vi "Begin.vi"(8 "error in":errorcluster) -> (0 "error out":errorcluster)   [LabVIEW 2017]
doc: "Called before other user functions, this VI is expected to open initial I/O refnums, load in file data, and do all program initialization. Notice that the <B>error out</B> terminal is simply used for data flow. Wiring it to other structures or subVIs ensures that this VI runs first."
uses:
  <vilib>/Rock Robotics/WPI/DriverStation/WPI_DriverStationRobotMode2.ctl
  <vilib>/Rock Robotics/WPI/Joystick/WPI_JoystickDeviceEnum.ctl
  <vilib>/Rock Robotics/WPI/ThirdParty/Phoenix-LabVIEW/Motor Controller/Controls/CTRE_Phoenix_MotorControl_ControlMode.ctl
  <vilib>/Rock Robotics/WPI/Solenoid/WPI_SolenoidChannel.ctl
  Robot Global Data.vi
  <vilib>/Rock Robotics/Network Tables/NT Write String Array.vi
  Public/Documents/Cross The Road Electronics/Phoenix-LabVIEW/Pigeon IMU/CTRE_PigeonIMU_Open_TalonSRX.vi
  <vilib>/Rock Robotics/WPI/Solenoid/WPI_SolenoidOpenDouble.vi
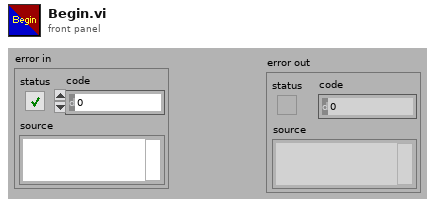
[diagram p1: front panel]
types:
  T1 = typedef "WPI_SolenoidChannel.ctl" = enum8{"Solenoid 0", "Solenoid 1", "Solenoid 2", "Solenoid 3", "Solenoid 4", "Solenoid 5", "Solenoid 6", "Solenoid 7", "Invalid"}
  T2 = typedef "CTRE_Phoenix_MotorControl_ControlMode.ctl" = u16
  T3 = typedef "WPI_JoystickDeviceEnum.ctl" = enum16{"USB 0", "USB 1", "USB 2", "USB 3", "USB 4", "USB 5"}
  T4 = typedef "WPI_DriverStationRobotMode2.ctl" = enum16{"Autonomous Disabled", "Autonomous Enabled", "Teleop Disabled", "Teleop Enabled", "Disconnected", "Finish", "Test Disabled", "Test Enabled", "Emergency Stopped"}
  T5 = typedef "WPI_MotorControlDeviceRef.ctl" = cluster{"DeviceStatus":errorcluster, "Type":T6, "PWM":cluster{"PWM Channel":T7, "DeadBand":T8}, "CAN":cluster{"Device Number":u8, "SetOutput VI Ref":variant, "GetOutput VI Ref":variant, "Enable VI Ref":variant, "Disable VI Ref":variant, "Data":variant}, "Invert":bool, "DIO PWM":cluster{"PWM \"Enable\" Channel":T7, "DIOChannel":T9, "PWM Rate":dbl}}
  T6 = typedef "WPI_MotorControlType.ctl" = enum16{"PWM", "CAN", "DIO PWM"}
  T7 = typedef "FPGA_DIOPWMChannel.ctl" = enum8{"PWM 0", "PWM 1", "PWM 2", "PWM 3", "PWM 4", "PWM 5", "PWM 6", "PWM 7", "PWM 8", "PWM 9", "PWM MXP 0", "PWM MXP 1", "PWM MXP 2", "PWM MXP 3", "PWM MXP 4", "PWM MXP 5", "PWM MXP 6", "PWM MXP 7", "PWM MXP 8", "PWM MXP 9", "Invalid"}
  T8 = typedef "WPI_PWMDeadband.ctl" = cluster{"Name":string, "maxPositivePwm":i32, "minPositivePwm":i32, "centerPwm":i32, "maxNegativePwm":i32, "minNegativePwm":i32, "angularRange":u16}
  T9 = typedef "FPGA_DIOChannel.ctl" = enum8{"DIO 0", "DIO 1", "DIO 2", "DIO 3", "DIO 4", "DIO 5", "DIO 6", "DIO 7", "DIO 8", "DIO 9", "DIO MXP 0", "DIO MXP 1", "DIO MXP 2", "DIO MXP 3", "DIO MXP 4", "DIO MXP 5", "DIO MXP 6", "DIO MXP 7", "DIO MXP 8", "DIO MXP 9", "DIO MXP 10", "DIO MXP 11", "DIO MXP 12", "DIO MXP 13", "DIO MXP 14", "DIO MXP 15", "SPI Port CS1", "SPI Port CS2", "SPI Port CS3", "SPI Port MISO", "SPI Port MOSI", "Invalid"}
  T10 = typedef "WPI_JoystickDevRef.ctl" = cluster{"Device":T3}
  T11 = typedef "CTRE_PigeonIMU_DeviceRef.ctl" = cluster{"DeviceStatus":errorcluster, "Device Number":u8, "Type":T12, "Device ID":u32, "Handle":u64, "UsageFrame":u32, "Library Path":path}
  T12 = typedef "CTRE_PigeonIMU_ConnectionType.ctl" = u32
  T13 = typedef "WPI_CompressorDevRef.ctl" = cluster{"DevStatus":errorcluster, "Pneumatics Control Module":u8}
  T14 = typedef "WPI_SolenoidDevRef.ctl" = cluster{"DevStatus":errorcluster, "Pneumatics Control Module":u8, "Forward Solenoid Channel":T1, "Reverse Solenoid Channel":T1}
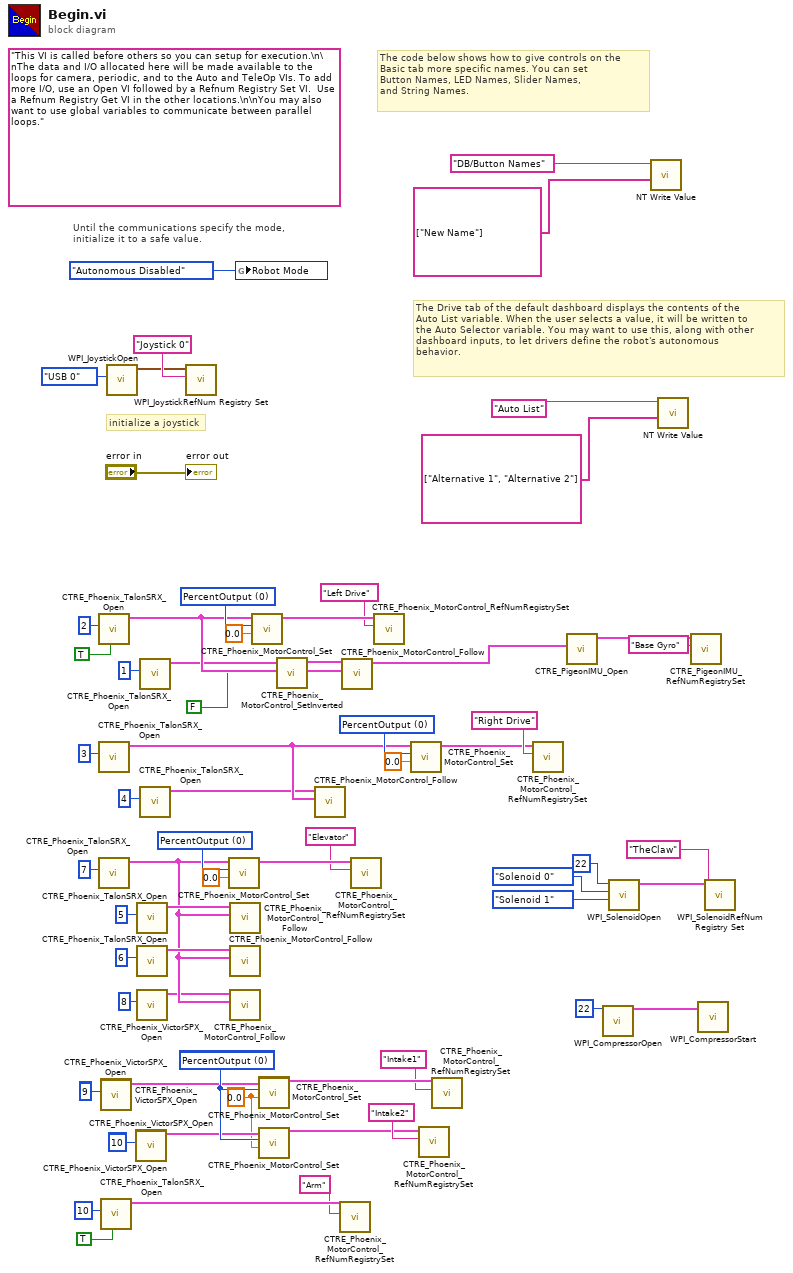
[diagram p0: block diagram]
diagram:
  w14 = 0.0 ("Output")
  w16 = T2 0 items=["PercentOutput"=0, "Position"=1, "Velocity"=2, "Current"=3, "Follower"=5, "MotionProfile"=6, "MotionMagic"=7, "MotionMagicArc"=8, "MotionProfileArc"=10, "Disabled"=15] ("Control Mode")
  w36 = T2 0 items=["PercentOutput"=0, "Position"=1, "Velocity"=2, "Current"=3, "Follower"=5, "MotionProfile"=6, "MotionMagic"=7, "MotionMagicArc"=8, "MotionProfileArc"=10, "Disabled"=15] ("Control Mode")
  w47 = T2 0 items=["PercentOutput"=0, "Position"=1, "Velocity"=2, "Current"=3, "Follower"=5, "MotionProfile"=6, "MotionMagic"=7, "MotionMagicArc"=8, "MotionProfileArc"=10, "Disabled"=15] ("Control Mode")
  w48 = T2 0 items=["PercentOutput"=0, "Position"=1, "Velocity"=2, "Current"=3, "Follower"=5, "MotionProfile"=6, "MotionMagic"=7, "MotionMagicArc"=8, "MotionProfileArc"=10, "Disabled"=15] ("Control Mode")
  w60 = T2 0 items=["PercentOutput"=0, "Position"=1, "Velocity"=2, "Current"=3, "Follower"=5, "MotionProfile"=6, "MotionMagic"=7, "MotionMagicArc"=8, "MotionProfileArc"=10, "Disabled"=15] ("Control Mode")
  (unwired) "This VI is called before others so you can setup for execution.\n\nThe data and I/O allocated here will be made available to the loops for camera, periodic, and to the Auto and TeleOp VIs. To add more I/O, use an Open VI followed by a Refnum Registry Set VI.  Use a Refnum Registry Get VI in the other locations.\n\nYou may also want to use global variables to communicate between parallel loops."
  # "The Drive tab of the default dashboard displays the contents of the\nAuto List variable. When the user selects a value, it will be written to\nthe Auto Selector variable. You may want to use this, along with other\ndashboard inputs, to let drivers define the robot's autonomous\nbehavior."
  # "The code below shows how to give controls on the\nBasic tab more specific names. You can set\nButton Names, LED Names, Slider Names,\nand String Names."
  # "initialize a joystick"
  # "Until the communications specify the mode,\ninitialize it to a safe value."
  n1 = call "CTRE_Phoenix_TalonSRX_Open.vi"("Invert"=TRUE, "Device Number"=u8 2) -> ("CAN Talon SRX Ref"=w56:T5)  [unwired: 8 in, 1 out]
  n2 = call "CTRE_Phoenix_TalonSRX_Open.vi"("Device Number"=u8 3) -> ("CAN Talon SRX Ref"=w29:T5)  [unwired: 9 in, 1 out]
  n3 = call "CTRE_Phoenix_TalonSRX_Open.vi"("Device Number"=u8 7) -> ("CAN Talon SRX Ref"=w38:T5)  [unwired: 9 in, 1 out]
  n4 = call "CTRE_Phoenix_VictorSPX_Open.vi"("Device Number"=u8 9) -> ("CAN Talon SRX Ref"=w32:T5)  [unwired: 9 in, 1 out]
  n5 = call "CTRE_Phoenix_VictorSPX_Open.vi"("Device Number"=u8 9) -> ("CAN Talon SRX Ref"=w33:T5)  [unwired: 9 in, 1 out]
  n6 = call "CTRE_Phoenix_TalonSRX_Open.vi"("Invert"=TRUE, "Device Number"=u8 10) -> ("CAN Talon SRX Ref"=w18:T5)  [unwired: 8 in, 1 out]
  n7 = call <vilib>:"WPI_JoystickOpen.vi"("JoystickDevice"=WPI_JoystickDeviceEnum."USB 0") -> ("JoystickDevRef"=w67:T10)  [unwired: 10 in]
  n8 = call "CTRE_Phoenix_VictorSPX_Open.vi"("Device Number"=u8 11) -> ("CAN Talon SRX Ref"=w15:T5)  [unwired: 9 in, 1 out]
  n9 = call "CTRE_Phoenix_VictorSPX_Open.vi"("Device Number"=u8 10) -> ()  [unwired: 9 in, 2 out]
  n10 = call "CTRE_Phoenix_TalonSRX_Open.vi"("Device Number"=u8 5) -> ("CAN Talon SRX Ref"=w43:T5)  [unwired: 9 in, 1 out]
  n11 = call "CTRE_Phoenix_TalonSRX_Open.vi"("Device Number"=u8 6) -> ("CAN Talon SRX Ref"=w40:T5)  [unwired: 9 in, 1 out]
  n12 = call "CTRE_Phoenix_VictorSPX_Open.vi"("Device Number"=u8 8) -> ("CAN Talon SRX Ref"=w20:T5)  [unwired: 9 in, 1 out]
  n13 = call "CTRE_Phoenix_TalonSRX_Open.vi"("Device Number"=u8 1) -> ("CAN Talon SRX Ref"=w27:T5)  [unwired: 9 in, 1 out]
  n14 = call "CTRE_Phoenix_TalonSRX_Open.vi"("Device Number"=u8 4) -> ("CAN Talon SRX Ref"=w25:T5)  [unwired: 9 in, 1 out]
  n15 = call <vilib>:"WPI_JoystickRefNum Registry Set.vi"("refnum name"="Joystick 0", "JoystickDevRef"=w67) -> ()  [unwired: 8 in, 2 out]
  n16 = call "CTRE_Phoenix_MotorControl_Set.vi"("Output"=0.0, "Control Mode"=w47, "PhoenixMotorControlDevRef"=w38) -> ("PhoenixMotorControlDevRef"=w42:T5)  [unwired: 7 in, 1 out]
  n17 = call "CTRE_Phoenix_MotorControl_Follow.vi"("Master Controller to Follow"=w38, "PhoenixMotorControlDevRef"=w43) -> ()  [unwired: 8 in, 2 out]
  n18 = call "CTRE_Phoenix_MotorControl_Follow.vi"("Master Controller to Follow"=w38, "PhoenixMotorControlDevRef"=w40) -> ()  [unwired: 8 in, 2 out]
  n19 = call "CTRE_Phoenix_MotorControl_Follow.vi"("Master Controller to Follow"=w38, "PhoenixMotorControlDevRef"=w20) -> ()  [unwired: 8 in, 2 out]
  n20 = global write "Robot Global Data.vi" "Robot Mode"(WPI_DriverStationRobotMode2."Autonomous Disabled" ("Robot Mode")) -> ()
  n21 = call "CTRE_Phoenix_MotorControl_Set.vi"("Output"=0.0, "Control Mode"=w60, "PhoenixMotorControlDevRef"=w56) -> ("PhoenixMotorControlDevRef"=w55:T5)  [unwired: 7 in, 1 out]
  n22 = call "CTRE_Phoenix_MotorControl_Set.vi"("Output"=w14, "Control Mode"=w16, "PhoenixMotorControlDevRef"=w32) -> ("PhoenixMotorControlDevRef"=w13:T5)  [unwired: 7 in, 1 out]
  n23 = call "CTRE_Phoenix_MotorControl_Set.vi"("Output"=0.0, "Control Mode"=w36, "PhoenixMotorControlDevRef"=w33) -> ()  [unwired: 7 in, 2 out]
  n24 = call "CTRE_Phoenix_MotorControl_Set.vi"("Output"=w14, "Control Mode"=w16, "PhoenixMotorControlDevRef"=w15) -> ("PhoenixMotorControlDevRef"=w10:T5)  [unwired: 7 in, 1 out]
  n25 = call <vilib>:"CTRE_Phoenix_MotorControl_SetInverted.vi"("Invert?"=FALSE ("Invert? Right"), "PhoenixMotorControlDevRef"=w27) -> ("PhoenixMotorControlDevRef"=w26:T5)  [unwired: 8 in, 1 out]
  n26 = call "CTRE_Phoenix_MotorControl_Follow.vi"("Master Controller to Follow"=w29, "PhoenixMotorControlDevRef"=w25) -> ()  [unwired: 8 in, 2 out]
  n27 = call "CTRE_Phoenix_MotorControl_RefNumRegistrySet.vi"("refnum name"="Arm", "PhoenixMotorControlDevRef"=w18) -> ()  [unwired: 8 in, 2 out]
  n28 = call "CTRE_Phoenix_MotorControl_Follow.vi"("Master Controller to Follow"=w56, "PhoenixMotorControlDevRef"=w26) -> ("PhoenixMotorControlDevRef"=w24:T5)  [unwired: 8 in, 1 out]
  n29 = call "CTRE_Phoenix_MotorControl_RefNumRegistrySet.vi"("refnum name"="Elevator", "PhoenixMotorControlDevRef"=w42) -> ()  [unwired: 8 in, 2 out]
  n30 = call "CTRE_Phoenix_MotorControl_RefNumRegistrySet.vi"("refnum name"="Left Drive", "PhoenixMotorControlDevRef"=w55) -> ()  [unwired: 8 in, 2 out]
  n31 = call "CTRE_Phoenix_MotorControl_Set.vi"("Output"=0.0, "Control Mode"=w48, "PhoenixMotorControlDevRef"=w29) -> ("PhoenixMotorControlDevRef"=w52:T5)  [unwired: 7 in, 1 out]
  n32 = call "CTRE_Phoenix_MotorControl_RefNumRegistrySet.vi"("refnum name"="Intake2", "PhoenixMotorControlDevRef"=w10) -> ()  [unwired: 8 in, 2 out]
  n33 = call "CTRE_Phoenix_MotorControl_RefNumRegistrySet.vi"("refnum name"="Intake1", "PhoenixMotorControlDevRef"=w13) -> ()  [unwired: 8 in, 2 out]
  n34 = call "CTRE_Phoenix_MotorControl_RefNumRegistrySet.vi"("refnum name"="Right Drive", "PhoenixMotorControlDevRef"=w52) -> ()  [unwired: 8 in, 2 out]
  n35 = call-poly "CTRE_PigeonIMU_Open.vi"("CAN Talon SRX Ref"=w24) -> ("PigeonIMUDevRef"=w23:T11)  [unwired: 9 in, 1 out]
  n36 = call <vilib>:"WPI_CompressorOpen.vi"("Pneumatics Control Module (0)"=u8 22) -> ("CompressorDevRef"=w1:T13)  [unwired: 13 in, 1 out]
  n37 = call-poly <vilib>:"WPI_SolenoidOpen.vi"("Reverse Solenoid Channel"=WPI_SolenoidChannel."Solenoid 1", "Forward Solenoid Channel"=WPI_SolenoidChannel."Solenoid 0", "Pneumatics Control Module (0)"=u8 22) -> ("SolenoidDevRef"=w8:T14)  [unwired: 7 in, 1 out]
  n38 = call-poly <vilib>:"NT Write Value.vi"("String Array"=string[] ["New Name"], "Name"="DB/Button Names") -> ()  [unwired: 9 in, 1 out]
  n39 = call-poly <vilib>:"NT Write Value.vi"("String Array"=string[] ["Alternative 1", "Alternative 2"], "Name"="Auto List") -> ()  [unwired: 9 in, 1 out]
  n40 = call "CTRE_PigeonIMU_RefNumRegistrySet.vi"("refnum name"="Base Gyro", "PigeonIMUDevRef"=w23) -> ()  [unwired: 8 in, 2 out]
  n41 = call <vilib>:"WPI_CompressorStart.vi"("CompressorDevRef"=w1) -> ()  [unwired: 9 in, 2 out]
  n42 = call <vilib>:"WPI_SolenoidRefNum Registry Set.vi"("refnum name"="TheClaw", "SolenoidDevRef"=w8) -> ()  [unwired: 8 in, 2 out]
  "error out" <- "error in"
